vi "Leitura_de_TXT.vi"() -> ()   [LabVIEW 2013]
uses:
  leitura de dados txt control.ctl
panel:
  out "Intepoled iluminants":dbl[][](array[numeric])
  out "Selected\nCMF":dbl[][](array[numeric])
  out "cmf Index":dbl
  out "CMFCols":i32
  out "CMFRows":i32
  out "CMF Table":string[][](array[string])
  in  "Color Matching Function":string(combo)
  out "ILCols":i32
  out "ILRows":i32
  out "XY Graph":T1(graph)
  out "GammaInterval":dbl[](array[numeric])
  out "NeedInterpolation?":bool
  out "Illuminant Tabel":string[][](array[string])
  out "Selected illuminant index":dbl
  in  "Select Illuminant":T2
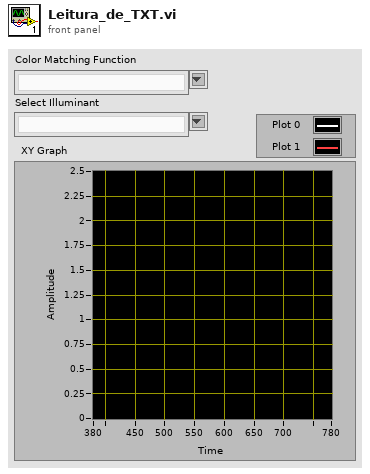
[diagram p1: front panel]
types:
  T1 = cluster{"GammaInterval":dbl[], "Interpolated":dbl[]}[]
  T2 = typedef "leitura de dados txt control.ctl" = string
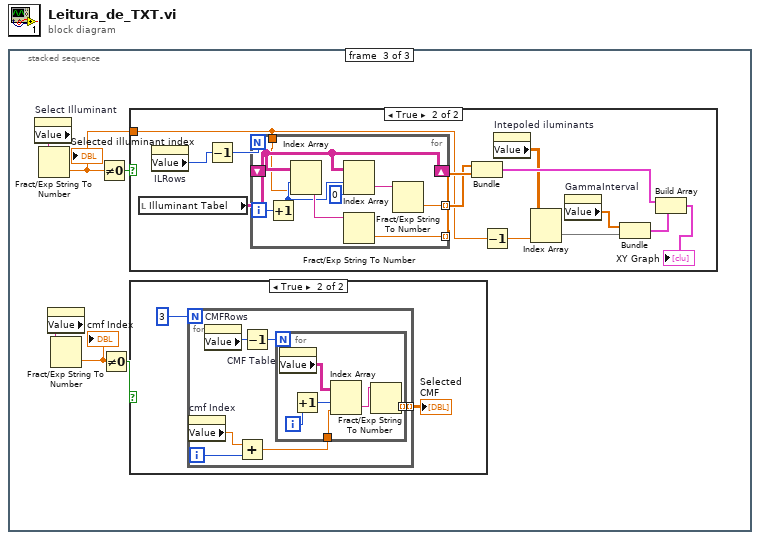
[diagram p0: block diagram]
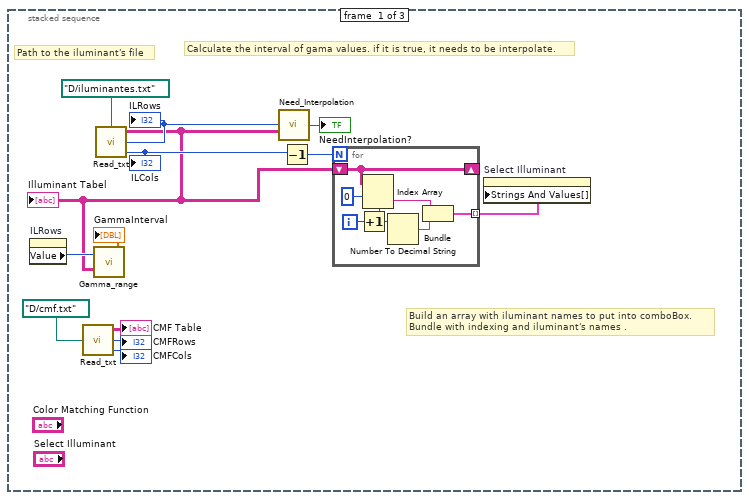
[diagram p2: hidden frame]
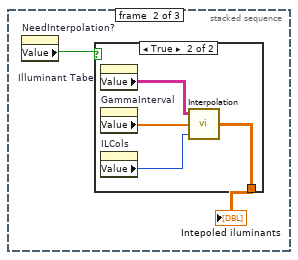
[diagram p3: hidden frame]
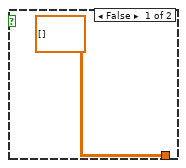
[diagram p4: hidden frame]
diagram:
  n1 = stacked-sequence {
    frame #0 {
      # "Calculate the interval of gama values. if it is true, it needs to be interpolate."
      # "Path to the iluminant's file"
      # "Build an array with iluminant names to put into comboBox.\nBundle with indexing and iluminant's names ."
      n2 = property on="ILRows" class="DigNum (strict)"() -> ("Value"=w6:i32)  [unwired: 2 in, 2 out]
      n3 = call "Read_txt.vi"("file path (dialog if empty)"=path "D:/cmf.txt") -> ("Elements"=→"CMF Table":string[][], "Rows"=→"CMFRows":i32, "Cols"=→"CMFCols":i32)
      n4 = call "Read_txt.vi"("file path (dialog if empty)"=path "D:/iluminantes.txt") -> ("Elements"=w5:string[][], "Rows"=w9:i32, "Cols"=w8:i32)
      "Illuminant Tabel" <- w5
      "ILRows" <- w9
      "ILCols" <- w8
      n5 = call "Gamma_range.vi"("Illuminant Table"=w5, "NumberOfRows"=w6) -> ("GammaInterval"=→"GammaInterval":dbl[])
      n6 = call "Need_Interpolation.vi"("Matrix with txt"=w5, "Number of Rows"=w9) -> ("isNotFive?"=→"NeedInterpolation?":bool)
      n7 = Decrement(x=w8) -> (x-1=w12:i32)
      n8 = for {
        N: w12 -> [_]
        shift-right: [w18] -> _
        shift-left: w5 -> [w18]
        tunnel: [w14] -> w13 mode=indexing
        i -> [w20]
        n9 = Increment(x=w20) -> (x+1=w17:i32)
        n10 = Index Array(array=w18, index (row)=0, index (col)=w17) -> (element=w15:string)
        n11 = Number To Decimal String(number=w17) -> (decimal integer string=w16:string)  [unwired: 1 in]
        n12 = Bundle("String"=w15, w16) -> (w14:cluster{"String":string, string})  [unwired: 1 in]
      }
      n13 = property on="Select Illuminant" class="CmbBox (strict)"("Strings And Values[]"=w13) -> ()  [unwired: 2 in, 2 out]
    }
    frame #1 {
      n14 = property on="NeedInterpolation?" class="Bool (strict)"() -> ("Value"=w22:bool)  [unwired: 2 in, 2 out]
      n15 = case shown="True" w22 {
        tunnel: [dbl[][] [] w24] -> w21
        frame False {
        }
        frame True {
          n16 = property on="Illuminant Tabel" class="Arr (strict)"() -> ("Value"=w27:string[][])  [unwired: 2 in, 2 out]
          n17 = property on="GammaInterval" class="Arr (strict)"() -> ("Value"=w26:dbl[])  [unwired: 2 in, 2 out]
          n18 = property on="ILCols" class="DigNum (strict)"() -> ("Value"=w25:i32)  [unwired: 2 in, 2 out]
          n19 = call "Interpolation.vi"("Number of Columns"=w25, "Lambda Interval"=w26, "Illuminants"=w27) -> ("Interpolated"=w24:dbl[][])
        }
      }
      "Intepoled iluminants" <- w21
    }
    frame #2 {
      n20 = property on="Select Illuminant" class="CmbBox (strict)"() -> ("Value"=w29:T2)  [unwired: 2 in, 2 out]
      n21 = Fract/Exp String To Number(string=w29) -> (number=w28:dbl)  [unwired: 3 in, 1 out]
      "Selected illuminant index" <- w28
      n22 = property on="Color Matching Function" class="CmbBox"() -> ("Value"=w31:string)  [unwired: 2 in, 2 out]
      n23 = Fract/Exp String To Number(string=w31) -> (number=w32:dbl)  [unwired: 3 in, 1 out]
      "cmf Index" <- w32
      n24 = Not Equal To 0?(x=w28) -> (x != 0?=w33:bool)
      n25 = Not Equal To 0?(x=w32) -> (x != 0?=w30:bool)
      n26 = case shown="True" w33 {
        tunnel: w28 -> [_ w52]
        frame False {
        }
        frame True {
          n27 = local read "Illuminant Tabel"() -> (w59:string[][])
          n28 = property on="ILRows" class="DigNum (strict)"() -> ("Value"=w50:i32)  [unwired: 2 in, 2 out]
          n29 = Decrement(x=w50) -> (x-1=w60:i32)
          n30 = for {
            N: w60 -> [_]
            shift-right: [w68] -> _
            shift-left: w59 -> [w68]
            tunnel: w52 -> [w61]
            tunnel: [w63] -> w58 mode=indexing
            tunnel: [w62] -> w57 mode=indexing
            i -> [w69]
            n31 = Increment(x=w69) -> (x+1=w64:i32)
            n32 = Index Array(array=w68, index (row)=w64, index (col)=w61) -> (element=w65:string)
            n33 = Index Array(array=w68, index (row)=w64, index (col)=0 ("disabled index (col)")) -> (element=w66:string)
            n34 = Fract/Exp String To Number(string=w65) -> (number=w63:dbl)  [unwired: 3 in, 1 out]
            n35 = Fract/Exp String To Number(string=w66) -> (number=w62:dbl)  [unwired: 3 in, 1 out]
          }
          n36 = Bundle(w57, w58) -> (w53:cluster{dbl[], dbl[]})  [unwired: 1 in]
          n37 = Decrement(x=w52) -> (x-1=w51:dbl)
          n38 = property on="Intepoled iluminants" class="Arr (strict)"() -> ("Value"=w49:dbl[][])  [unwired: 2 in, 2 out]
          n39 = Index Array(array=w49, index (col)=w51) -> (element=w54:dbl[])  [unwired: 1 in]
          n40 = property on="GammaInterval" class="Arr (strict)"() -> ("Value"=w48:dbl[])  [unwired: 2 in, 2 out]
          n41 = Bundle("Value"=w48, "Value"=w54) -> (w55:cluster{"Value":dbl[], "Value":dbl[]})  [unwired: 1 in]
          n42 = Build Array(w53, w55) -> (→"XY Graph":cluster{"Value":dbl[], "Value":dbl[]}[])
        }
      }
      n43 = case shown="True" w30 {
        frame False {
        }
        frame True {
          n44 = for {
            N: 3 -> [_]
            tunnel: [w38] -> w34 mode=indexing
            i -> [w40]
            n45 = property on="cmf Index" class="DigNum (strict)"() -> ("Value"=w41:dbl)  [unwired: 2 in, 2 out]
            n46 = property on="CMFRows" class="DigNum (strict)"() -> ("Value"=w37:i32)  [unwired: 2 in, 2 out]
            n47 = Add(x=w41, y=w40) -> (x+y=w39:dbl)
            n48 = Decrement(x=w37) -> (x-1=w36:i32)
            n49 = for {
              N: w36 -> [_]
              tunnel: w39 -> [w46]
              tunnel: [w42] -> w38 mode=indexing
              i -> [w45]
              n50 = property on="CMF Table" class="Arr (strict)"() -> ("Value"=w47:string[][])  [unwired: 2 in, 2 out]
              n51 = Increment(x=w45) -> (x+1=w44:i32)
              n52 = Index Array(array=w47, index (row)=w44, index (col)=w46) -> (element=w43:string)
              n53 = Fract/Exp String To Number(string=w43) -> (number=w42:dbl)  [unwired: 3 in, 1 out]
            }
          }
          "Selected\nCMF" <- w34
        }
      }
    }
  }
